vi "File Read.vi"(4 "file path":path) -> (1 "data":string)   [LabVIEW 2016]
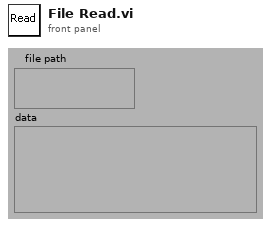
[diagram p1: front panel]
types:
  T1 = enum16{"open", "open or create", "create or replace", "create", "open (read only)"}
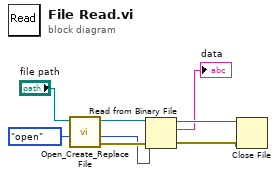
[diagram p0: block diagram]
diagram:
  n1 = call <vilib>:"Open_Create_Replace File.vi"("function (open:0)"=T1."open", "file path"="file path") -> ("error out"=w6:errorcluster, "file size (bytes)"=w1:i32, "refnum"=w8:refnum<file>)  [unwired: 6 in, 1 out]
  n2 = Read from Binary File(8:w6, 10:w1, 11:w8) -> (0:w5:errorcluster, 2:→"data":string, 3:w7:refnum<file>)  [unwired: 3 in, 1 out]
  n3 = Close File(refnum=w7, error in=w5) -> ()  [unwired: 2 out]
